vi "[FPGA] DeltaSig Main V3.vi"() -> ()   [LabVIEW 2015]
doc: "This VI provides a template for customizing a waveform acquisition using delta-sigma based NI C Series analog input smodules."
uses:
  <vilib>/LabVIEW Targets/FPGA/cRIO/shared/nicrio_ModuleControls/nicrio_cRIO-9234_ConfigModeRing.ctl
  <vilib>/rvi/Emulation/niFpgaGetClockAttributes.vi
  <vilib>/rvi/Emulation/niFpgaSctlEmulationGetInTimedLoop.vi
  <vilib>/rvi/Emulation/niFpgaEmulationReportErrorSimple.vi
  <vilib>/LabVIEW Targets/FPGA/cRIO/shared/nicrio_DsaDataRateApi/_nicrio_9234GetDataRate131.vi
  <vilib>/rvi/Emulation/niFpgaProcessEmulError.vi
  <vilib>/rvi/eio/common/nirviEmuTemplatePropertySet_errors.vi
  <vilib>/rvi/eio/common/nirviEmuTemplateMethod_errors.vi
  <vilib>/rvi/interface/RandomDataEmulation/niFpgaRandomDataHandleErrors.vi
  <vilib>/rvi/Emulation/niFpgaCriticalErrorInLSC.vi
  <vilib>/eio/EIOPropertyNode/EIOPropertyNode.xnode
  <vilib>/LabVIEW Targets/FPGA/cRIO/shared/nicrio_ModuleControls/nicrio_cRIO-9234_DataRatesRing2.ctl
  <vilib>/eio/EIONode/EIONode.xnode
  <vilib>/rvi/DataTransferAndStorage/Container/XNode/niFpgaContainer.xnode
  <vilib>/rvi/interface/RandomDataEmulation/nirviRandomDataFpgaReadWriteTemplate.vi
  <vilib>/rvi/eio/common/nirviEmuTemplatePropertyGet_errors.vi
  <vilib>/rvi/eio/common/nirviEmuTemplatePropertyGet_noerrors.vi
  <vilib>/rvi/eio/common/nirviEmuTemplatePropertySet_noerrors.vi
panel:
  in  "Array Input Config":T1[](array[typedef])=[0, 0, 0, 0] items=["AC Coupled", "DC Coupled", "IEPE AC Coupled"]
  out "oclk freq":u32
  out "oclk div":u32
  out "oclk mult":u32
  in  "data rate (S/s)":u32
  in  "Chan Scale Array":sgl[](array[numeric])=[0.0, 0.0, 0.0, 0.0, 0.0, 0.0, 0.0, 0.0, 0.0, 0.0, 0.0, 0.0, 0.0, 0.0, 0.0, 0.0, 0.0, 0.0, 0.0, 0.0, 0.0, 0.0, 0.0, 0.0, 0.0, 0.0, 0.0, 0.0, 0.0, 0.0, 0.0, 0.0, 0.0, 0.0, 0.0, 0.0, 0.0, 0.0, 0.0, 0.0]
  out "Chan Count":bool
  out "Acq Loop Ticks":u32
  out "FPGA Error":errorcluster
  out "Module Underflow":bool
  out "Finished":bool
  in  "Number of Channels":i32=4
  in  "Samps per Chan [Finite]":i32=5120
  out "First Read":bool
  in  "Acquisition Type":enum16{"Finite Samples", "Continuous Samples"}(ring)
  out "DMA FIFO Full":bool
  in  "stop":bool
  # "Array size fixed at 40\nelements but may be \nexpanded if needed"
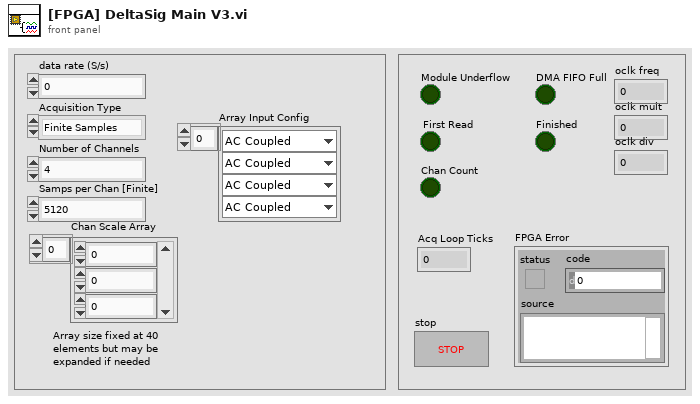
[diagram p1: front panel]
types:
  T1 = typedef "nicrio_cRIO-9234_ConfigModeRing.ctl" = u8
  T2 = typedef "nicrio_cRIO-9234_DataRatesRing2.ctl" = u8
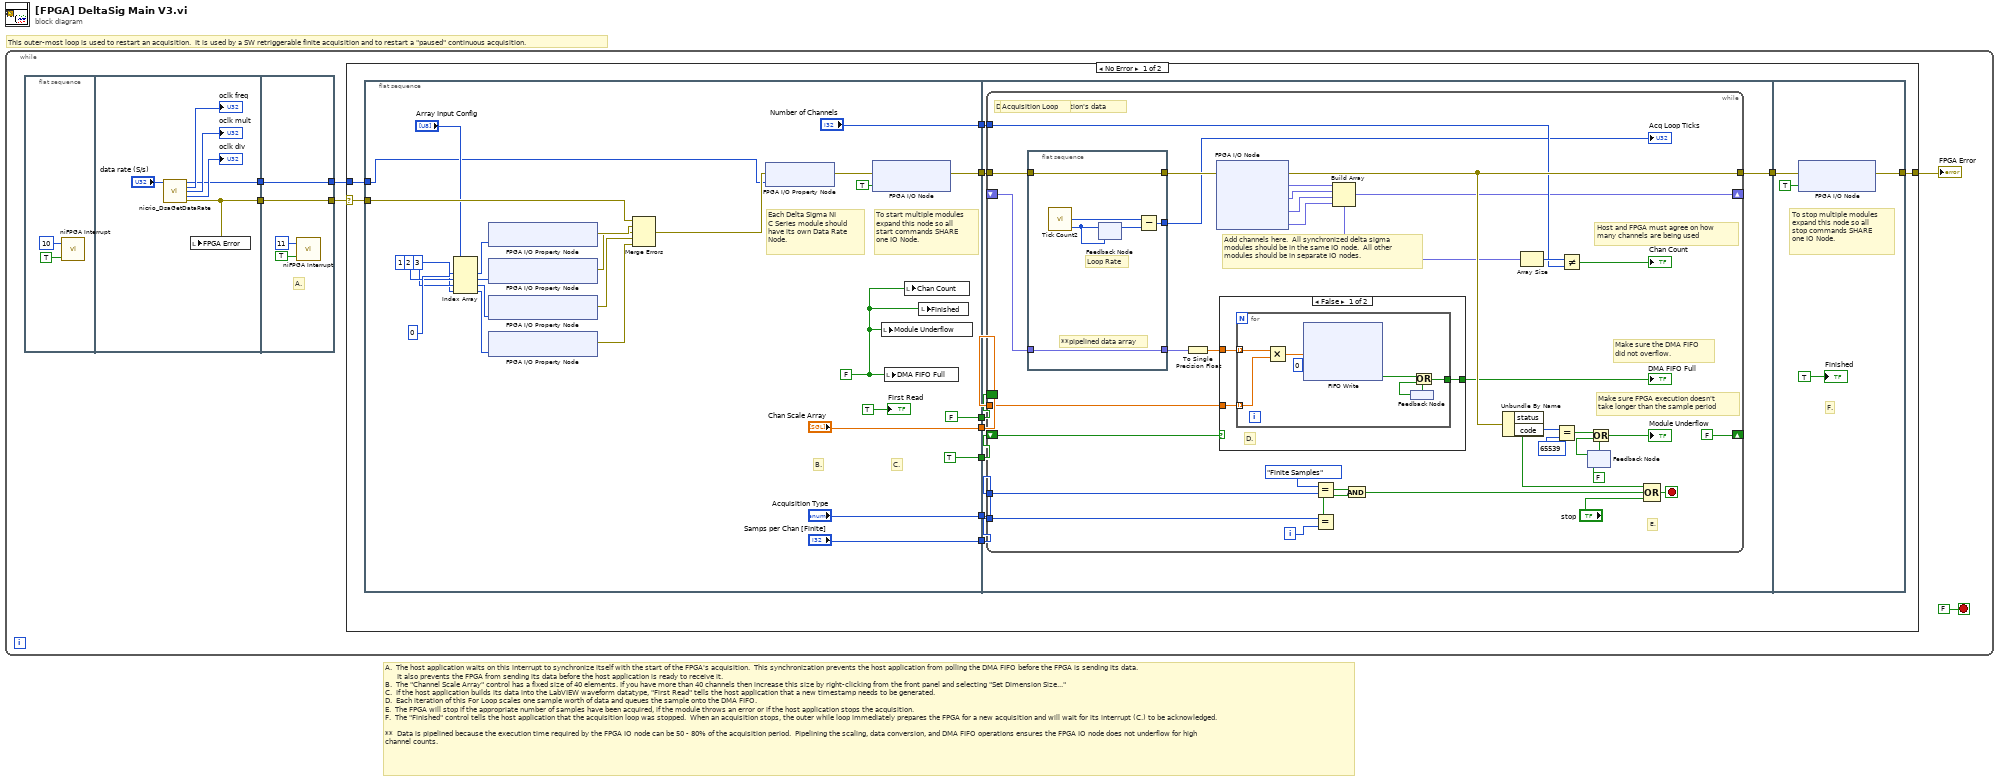
[diagram p0: block diagram]
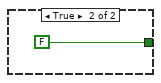
[diagram p2: hidden frame]
diagram:
  # "A.  The host application waits on this interrupt to synchronize itself with the start of the FPGA's acquisition.  This synchronization prevents the host application from polling the DMA FIFO before the FPGA is sending its data.\n      It also prevents the FPGA from sending its data before the host application is ready to receive it.\nB.  The \"Channel Scale Array\" control has a fixed size of 40 elements. If you have more than 40 channels then increase this size by right-clicking from the front panel and selecting \"Set Dimension Size...\"\nC.  If the host application builds its data into the LabVIEW waveform datatype, \"First Read\" tells the host application that a new timestamp needs to be generated.\nD.  Each iteration of this For Loop scales one sample worth of data and queues the sample onto the DMA FIFO.  \nE.  The FPGA will stop if the appropriate number of samples have been acquired, if the module throws an error or if the host application stops the acquisition.  \nF.  The \"Finished\" control tells the host application that the acquisition loop was stopped.  When an acquisition stops, the outer while loop immediately prepares the FPGA for a new acquisition and will wait for its interrupt (C.) to be acknowledged.\n\n**  Data is pipelined because the execution time required by the FPGA IO node can be 50 - 80% of the acquisition period.  Pipelining the scaling, data conversion, and DMA FIFO operations ensures the FPGA IO node does not underflow for high\nchannel counts."
  # "This outer-most loop is used to restart an acquisition.  It is used by a SW retriggerable finite acquisition and to restart a \"paused\" continuous acquisition."
  n1 = while {
    stop <- FALSE stop-if-true
    n2 = flat-sequence {
      tunnel: [w10] -> w2
      tunnel: [w11] -> w1
      tunnel: [w18] -> w3
      tunnel: [w15] -> w4
      tunnel: w2 -> [w15]
      tunnel: w1 -> [w18]
      frame #0 {
        n3 = call <vilib>:"niFPGA Interrupt.vi"("Wait Until Cleared (F)"=TRUE ("Wait Until Cleared"), "IRQ Number (0)"=u8 10 ("IRQ Number")) -> ()  [unwired: 1 in]
      }
      frame #1 {
        n4 = call-poly <vilib>:"nicrio_DsaGetDataRate.vi"("data rate (S/s)"="data rate (S/s)") -> ("data rate"=w11:T2, "oclk freq"=→"oclk freq":u32, "oclk mult"=→"oclk mult":u32, "oclk div"=→"oclk div":u32, "error out"=w10:errorcluster)  [unwired: 10 in]
        n5 = local write "FPGA Error"(w10) -> ()
      }
      frame #2 {
        # "A."
        n6 = call <vilib>:"niFPGA Interrupt.vi"("Wait Until Cleared (F)"=TRUE ("Wait Until Cleared"), "IRQ Number (0)"=u8 11 ("IRQ Number")) -> ()  [unwired: 1 in]
      }
    }
    n7 = case shown="No Error" w4 {
      selector: w4 -> [w19 w120]
      tunnel: [w21 w120] -> w5
      tunnel: w3 -> [w20 _]
      frame No Error {
        n8 = flat-sequence {
          tunnel: [w56] -> w29
          tunnel: ["Chan Scale Array"] -> w28
          tunnel: ["Acquisition Type"] -> w27
          tunnel: ["Samps per Chan [Finite]"] -> w26
          tunnel: ["Number of Channels"] -> w25
          tunnel: [TRUE ("t")] -> w24
          tunnel: [FALSE] -> w23
          tunnel: w20 -> [w30]
          tunnel: w19 -> [w37]
          tunnel: w29 -> [w63]
          tunnel: w28 -> [w62]
          tunnel: w27 -> [w60]
          tunnel: w26 -> [w59]
          tunnel: w25 -> [w64]
          tunnel: w24 -> [w61]
          tunnel: [w58] -> w22
          tunnel: w23 -> [w57]
          tunnel: w22 -> [w117]
          tunnel: [w116] -> w21
          frame #0 {
            w53 = FALSE ("Module Underflow")
            # "To start multiple modules\nexpand this node so all\nstart commands SHARE\none IO Node."
            # "C."
            # "B."
            # "Each Delta Sigma NI \nC Series module should \nhave its own Data Rate \nNode."
            n9 = Index Array(array="Array Input Config", index #1=0 ("index"), index #2=1 ("index"), index #3=2 ("index"), index #4=3 ("index")) -> (element #1=w44:T1, element #2=w43:T1, element #3=w42:T1, element #4=w41:T1)
            n10 = xnode "FPGA I/O Property Node"("Input Configuration"=w44) -> ("error out"=w36:errorcluster)  [unwired: 2 in, 1 out]
            n11 = xnode "FPGA I/O Property Node"("Input Configuration"=w43) -> ("error out"=w35:errorcluster)  [unwired: 2 in, 1 out]
            n12 = xnode "FPGA I/O Property Node"("Input Configuration"=w42) -> ("error out"=w34:errorcluster)  [unwired: 2 in, 1 out]
            n13 = xnode "FPGA I/O Property Node"("Input Configuration"=w41) -> ("error out"=w33:errorcluster)  [unwired: 2 in, 1 out]
            n14 = Merge Errors(w37, w36, w35, w34, w33) -> (w32:errorcluster)
            n15 = xnode "FPGA I/O Property Node"("error in"=w32, "Data Rate"=w30) -> ("error out"=w52:errorcluster)  [unwired: 1 in, 1 out]
            n16 = xnode "FPGA I/O Node"("error in"=w52, "Mod1/Start"=TRUE) -> ("error out"=w56:errorcluster)  [unwired: 1 in, 1 out]
            n17 = local write "Module Underflow"(w53) -> ()
            n18 = local write "DMA FIFO Full"(w53) -> ()
            n19 = local write "Chan Count"(w53) -> ()
            n20 = local write "Finished"(w53) -> ()
            "First Read" <- TRUE ("First Read")
          }
          frame #1 {
            n21 = while {
              tunnel: w63 -> [w87]
              tunnel: [w92] -> w58
              tunnel: w60 -> [w94]
              tunnel: w59 -> [w93]
              shift-right: [w67] -> _
              shift-left: _ -> [w80]
              tunnel: w64 -> [w89]
              tunnel: w62 -> [w81]
              shift-right: [FALSE ("t")] -> _
              shift-left: w61 -> [w79]
              border: w57 -> [_]
              i -> [w77]
              stop <- w97 stop-if-true
              # "Add channels here.  All synchronized delta sigma\nmodules should be in the same IO node.  All other\nmodules should be in separate IO nodes."
              # "Do not DMA first iteration's data"
              # "Acquisition Loop"
              # "E."
              # "Host and FPGA must agree on how \nmany channels are being used"
              # "Make sure the DMA FIFO\ndid not overflow."
              # "Make sure FPGA execution doesn't\ntake longer than the sample period"
              n22 = flat-sequence {
                tunnel: [w115] -> w86
                tunnel: w87 -> [w115]
                tunnel: [w112] -> w85
                tunnel: w80 -> [w111]
                tunnel: [w111] -> w66
                frame #0 {
                  # "**pipelined data array"
                  # "Loop Rate"
                  n23 = call "Tick Count2"() -> ("Tick Count(Ticks)"=w114:u32)
                  n24 = feedback-in #1(w114) -> ()
                  n25 = feedback #1(w114) -> (w113:u32)
                  n26 = Subtract(x=w114, y=w113) -> (x-y=w112:u32)
                }
              }
              n27 = To Single Precision Float(number=w66) -> (single precision float=w65:sgl[])
              n28 = xnode "FPGA I/O Node"("error in"=w86) -> ("error out"=w92:errorcluster, "Mod1/AI0"=w84:fxp<+/-,24,4>, "Mod1/AI1"=w76:fxp<+/-,24,4>, "Mod1/AI2"=w83:fxp<+/-,24,4>, "Mod1/AI3"=w82:fxp<+/-,24,4>)  [unwired: 4 in, 4 out]
              n29 = case shown="False" w79 {
                tunnel: [w102 FALSE] -> w91
                tunnel: w81 -> [w101 _]
                tunnel: w65 -> [w100 _]
                frame False {
                  # "D."
                  n30 = for {
                    tunnel: [w107] -> w102
                    tunnel: w100 -> [w105] mode=indexing
                    tunnel: w101 -> [w104] mode=indexing
                    n31 = Multiply(x=w105, y=w104) -> (x*y=w103:sgl)
                    n32 = xnode ("FIFO Write")("Element"=w103, "Timeout"=0) -> ("Timed Out?"=w109:bool)  [unwired: 1 in, 1 out]
                    n33 = feedback #2() -> (w108:bool)
                    n34 = Or(x=w109, y=w108) -> (x .or. y?=w107:bool)
                    n35 = feedback-in #2(w107) -> ()
                  }
                }
                frame True {
                }
              }
              "DMA FIFO Full" <- w91
              n36 = Equal?(x=enum16{"Finite Samples", "Continuous Samples"}."Finite Samples" ("y"), y=w94) -> (x = y?=w70:bool)
              n37 = Equal?(x=w93, y=w77) -> (x = y?=w69:bool)
              n38 = Build Array(w84, w76, w83, w82) -> (w67:fxp<+/-,24,4>[])
              n39 = And(x=w70, y=w69) -> (x .and. y?=w68:bool)
              n40 = Unbundle By Name(w92) -> ("status"=w75:bool, "code"=w95:i32)
              n41 = Array Size(array=w67) -> (size(s)=w90:i32)
              n42 = Equal?(x=w95, y=65539) -> (x = y?=w72:bool)
              n43 = Not Equal?(x=w90, y=w89) -> (x != y?=→"Chan Count":bool)
              n44 = feedback #3(FALSE) -> (w74:bool)
              n45 = Or(x=w72, y=w74) -> (x .or. y?=w71:bool)
              "Module Underflow" <- w71
              n46 = feedback-in #3(w71) -> ()
              n47 = Compound Arithmetic op=OR(w75, w68, "stop") -> (w97:bool)
              "Acq Loop Ticks" <- w85
            }
          }
          frame #2 {
            # "To stop multiple modules\nexpand this node so all\nstop commands SHARE\none IO Node."
            # "F."
            n48 = xnode "FPGA I/O Node"("error in"=w117, "Mod1/Stop"=TRUE) -> ("error out"=w116:errorcluster)  [unwired: 1 in, 1 out]
            "Finished" <- TRUE ("Finished")
          }
        }
      }
      frame Error {
      }
    }
    "FPGA Error" <- w5
  }
